vi "LIREETECRIREMODBUSLOGO.vi"(10 "coils to write":bool[](array[boolean])) -> (3 "coils":bool[](array[boolean]), 11 "I1 TO I8":bool[](array[boolean]))   [LabVIEW 2021]
uses:
  <vilib>/NI/Modbus Library/API/Wrapper/Create TCP Master.vi
  <vilib>/NI/Modbus Library/API/Master/Modbus Master.lvclass
  <vilib>/NI/Modbus Library/API/Wrapper/API Main.lvlib
panel:
  in  "error in":errorcluster
  out "error out":errorcluster
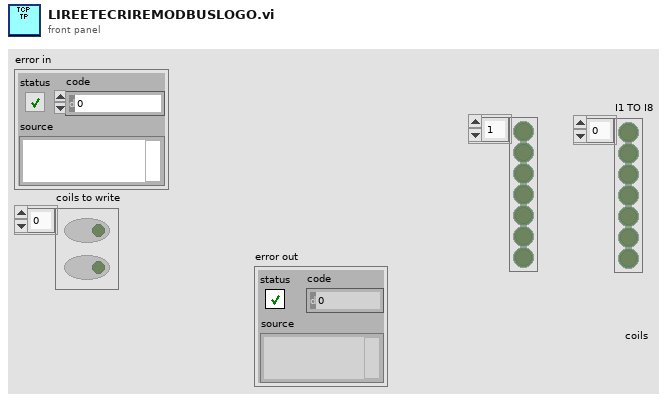
[diagram p1: front panel]
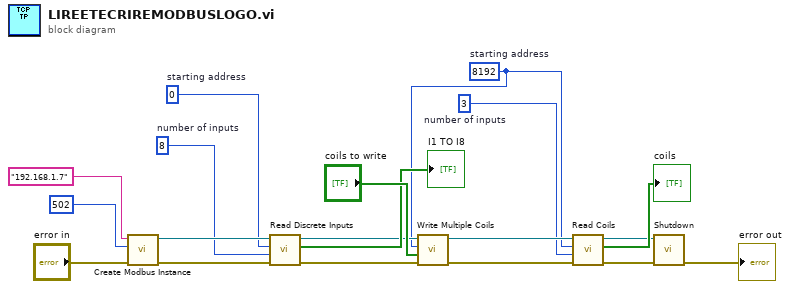
[diagram p0: block diagram]
diagram:
  w5 = u16 8  # number of inputs
  w4 = u16 0  # starting address
  w3 = u16 3  # number of inputs
  w6 = u16 8192  # starting address
  n1 = call-poly <vilib>:"Create Modbus Instance.vi"("error in"="error in", "port (502)"=u16 502, "address"="192.168.1.7") -> ("error out"=w14:errorcluster, "TCP master instance"=w13:refnum<class "Modbus Master.lvclass">)  [unwired: 7 in]
  n2 = call-dynamic "Read Discrete Inputs.vi"("error in"=w14, "number of inputs"=w5, "starting address"=w4, "Modbus master in"=w13) -> ("error out"=w11:errorcluster, "discrete inputs"=→"I1 TO I8":bool[], "Modbus master out"=w12:refnum<class "Modbus Master.lvclass">)  [unwired: 5 in]
  n3 = call-dynamic "Write Multiple Coils.vi"("error in"=w11, "coils to write"="coils to write", "starting address"=w6, "Modbus master in"=w12) -> ("error out"=w9:errorcluster, "Modbus master out"=w10:refnum<class "Modbus Master.lvclass">)  [unwired: 6 in]
  n4 = call-dynamic "Read Coils.vi"("error in"=w9, "number of inputs"=w3, "starting address"=w6, "Modbus master in"=w10) -> ("error out"=w16:errorcluster, "coils"=→"coils":bool[], "Modbus master out"=w15:refnum<class "Modbus Master.lvclass">)  [unwired: 5 in]
  n5 = call-dynamic "Shutdown.vi"("error in"=w16, "Modbus master in"=w15) -> ("error out"=→"error out":errorcluster)  [unwired: 9 in]
